vi "Backout on Error.vi"(8 "error in (no error)":errorcluster, 11 "QControl Creation in":refnum<class "QControl Creation.lvclass">) -> (0 "error out":errorcluster, 3 "QControl Creation out":refnum<class "QControl Creation.lvclass">)   [LabVIEW 2015, in "QControl Creation.lvclass"]
doc: "<b> </b> <b> </b>\n©2016 Q Software Innovations, LLC (QSI)\nwritten by Quentin Alldredge\nproduced in LabVIEW 2015\n\nsupport@qsoftwareinnovations.com\nwww.qsoftwareinnovations.com\n\nAll rights reserved.\n\nRedistribution and use in source and binary forms, with or without modification, are permitted provided that the following conditions are met:\n\n * Redistributions of source code must retain the above copyright notice, this list of conditions and the following disclaimer.\n * Redistributions in binary form must reproduce the above copyright notice, this list of conditions and the following disclaimer in the documentation and/or other materials provided with the distribution.\n * Neither the name of Q Software Innovations, LLC. nor the names of its contributors may be used to endorse or promote products derived from this software without specific prior written permission.\n\nTHIS SOFTWARE IS PROVIDED BY THE COPYRIGHT HOLDERS AND CONTRIBUTORS \"AS IS\" AND ANY EXPRESS OR IMPLIED WARRANTIES, INCLUDING, BUT NOT LIMITED TO, THE IMPLIED WARRANTIES OF MERCHANTABILITY AND FITNESS FOR A PARTICULAR PURPOSE ARE DISCLAIMED. IN NO EVENT SHALL THE COPYRIGHT OWNER OR CONTRIBUTORS BE LIABLE FOR ANY DIRECT, INDIRECT, INCIDENTAL, SPECIAL, EXEMPLARY, OR CONSEQUENTIAL DAMAGES (INCLUDING, BUT NOT LIMITED TO, PROCUREMENT OF SUBSTITUTE GOODS OR SERVICES; LOSS OF USE, DATA, OR PROFITS; OR BUSINESS INTERRUPTION) HOWEVER CAUSED AND ON ANY THEORY OF LIABILITY, WHETHER IN CONTRACT, STRICT LIABILITY, OR TORT (INCLUDING NEGLIGENCE OR OTHERWISE) ARISING IN ANY WAY OUT OF THE USE OF THIS SOFTWARE, EVEN IF ADVISED OF THE POSSIBILITY OF SUCH DAMAGE."
uses:
  QControl Creation.lvclass
  QControl Creation.lvclass/QControl Creation.ctl
  New QControl Info/New QControl Info.lvclass/New QControl Info.ctl
  New QControl Info/Read New Class Path.vi
  New QControl Info/New QControl Info.lvclass
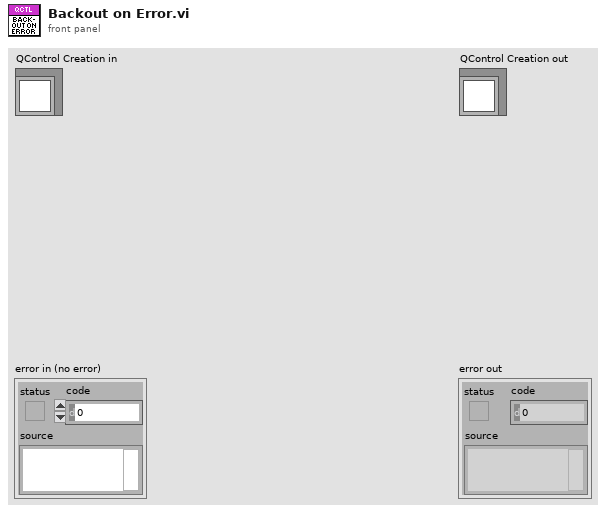
[diagram p1: front panel]
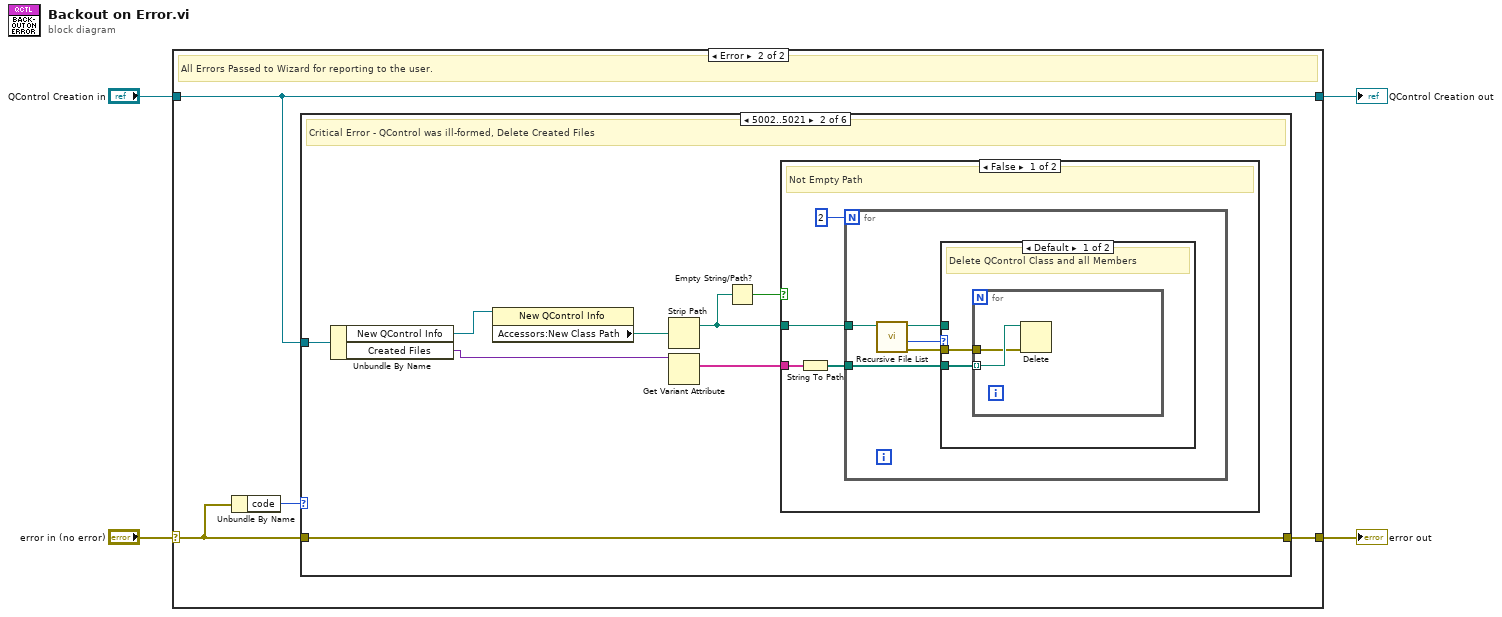
[diagram p0: block diagram]
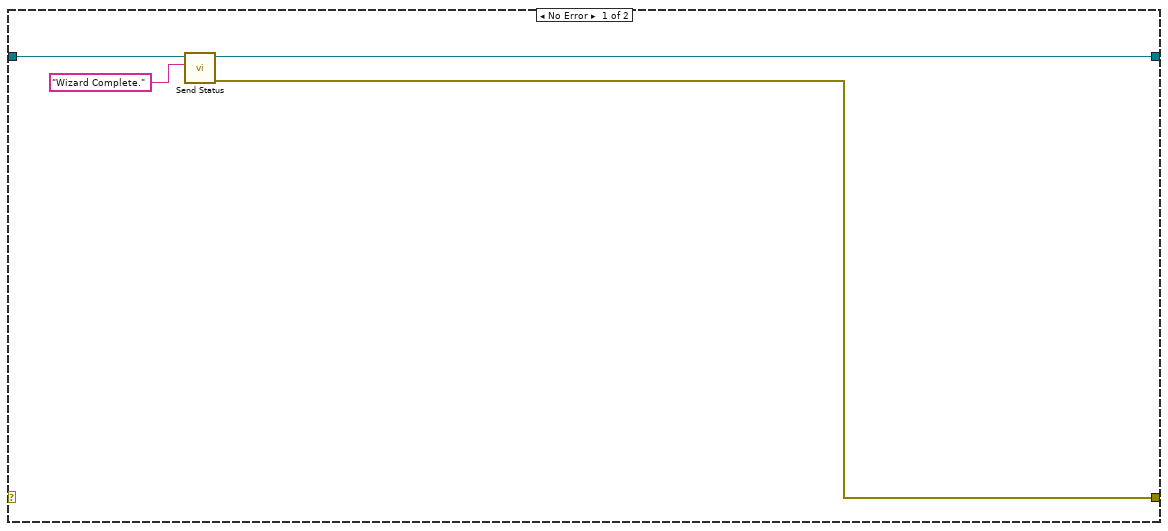
[diagram p2: hidden frame]
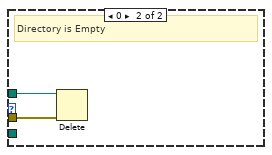
[diagram p4: hidden frame]
diagram:
  n1 = case shown="Error" "error in (no error)" {
    selector: "error in (no error)" -> [_ w11]
    tunnel: [w5 w12] -> w4
    tunnel: [w7 w10] -> w2
    tunnel: "QControl Creation in" -> [w8 w10]
    frame No Error {
      n2 = call "Send Status.vi"("Status"="Wizard Complete." ("Value"), "QControl Creation in"=w8) -> ("error out (dup)"=w5:errorcluster, "QControl Creation (dup)"=w7:refnum<class "QControl Creation.lvclass">)  [unwired: 8 in]
    }
    frame Error {
      # "All Errors Passed to Wizard for reporting to the user."
      n3 = Unbundle By Name(w11) -> ("code"=w9:i32)
      n4 = case shown="5002..5021" w9 {
        tunnel: [w13 w21 w37 w38 w39 w40] -> w12
        tunnel: w11 -> [w13 w21 w37 w38 w39 w40]
        tunnel: w10 -> [_ w20 _ _ _ _]
        frame Default {
          # "Other Errors"
        }
        frame 5002..5021 {
          # "Critical Error - QControl was ill-formed, Delete Created Files"
          n5 = Unbundle By Name(w20) -> ("New QControl Info"=w17:refnum<data-value>, "Created Files"=w19:variant)
          n6 = property class="New QControl Info"(reference=w17) -> ("Accessors:New Class Path"=w14:path)  [unwired: 1 in, 2 out]
          n7 = Strip Path(path=w14) -> (stripped path=w16:path)  [unwired: 1 out]
          n8 = Get Variant Attribute(Variant=w19) -> (names=w18:string[])  [unwired: 3 in, 3 out]
          n9 = Empty String/Path?(string/path=w16) -> (empty?=w15:bool)
          n10 = case shown="False" w15 {
            tunnel: w18 -> [w24 _]
            tunnel: w16 -> [w22 _]
            frame False {
              # "Not Empty Path"
              n11 = String To Path(string=w24) -> (path=w23:path[])
              n12 = for {
                N: 2 -> [_]
                tunnel: w22 -> [w29]
                tunnel: w23 -> [w30]
                n13 = call <vilib>:"Recursive File List.vi"("Folder Path"=w29) -> ("error out"=w26:errorcluster, "Number of Files"=w28:i32, "dup Folder Path"=w27:path)  [unwired: 6 in, 2 out]
                n14 = case shown="Default" w28 {
                  tunnel: w27 -> [_ w36]
                  tunnel: w26 -> [w31 w35]
                  tunnel: w30 -> [w32 _]
                  frame Default {
                    # "Delete QControl Class and all Members"
                    n15 = for {
                      tunnel: w32 -> [w34] mode=indexing
                      tunnel: w31 -> [w33]
                      n16 = Delete(path (use dialog)=w34, error in=w33) -> ()  [unwired: 3 in, 3 out]
                    }
                  }
                  frame 0 {
                    # "Directory is Empty"
                    n17 = Delete(path (use dialog)=w36, error in=w35) -> ()  [unwired: 3 in, 3 out]
                  }
                }
              }
            }
            frame True {
              # "Empty Path"
            }
          }
        }
        frame 5022 {
          # "Cosmetic Error - Error occured while applying class icon, Keep QControl, Inform User"
        }
        frame 5023 {
          # "Project Error - Could not Add to Project, Keep QControl, Inform User"
        }
        frame 5024 {
          # "Open Class Error - Could not Open QControl Class, Keep QControl, Inform User"
        }
        frame 5025..5031 {
          # "Prechecks - QControl creation is stopped before it started"
        }
      }
    }
  }
  "error out" <- w4
  "QControl Creation out" <- w2
